vi "3D_to_Pixels.vi"(0 "X_3D":dbl, 5 "Y_3D":dbl, 7 "Z_3D":dbl, 11 "Distance_3D":dbl) -> (4 "X_pixels":dbl, 6 "Y_pixels":dbl, 8 "Z_pixels":dbl, 15 "Distance_pixels":dbl)   [LabVIEW 2011]
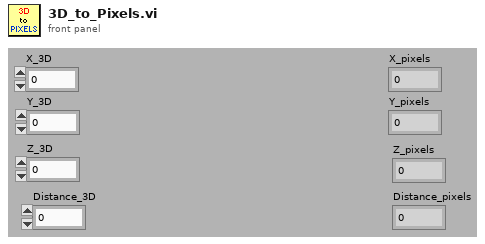
[diagram p1: front panel]
types:
  T1 = typedef "LVAllMonitorsDisplayTypeDef.ctl" = cluster{"Bounds":cluster{"Left":i16, "Top":i16, "Right":i16, "Bottom":i16}, "Depth":i16}[]
  T2 = cluster{"Bounds":cluster{"Left":i16, "Top":i16, "Right":i16, "Bottom":i16}, "Depth":i16}
  T3 = cluster{"Left":i16, "Top":i16, "Right":i16, "Bottom":i16}
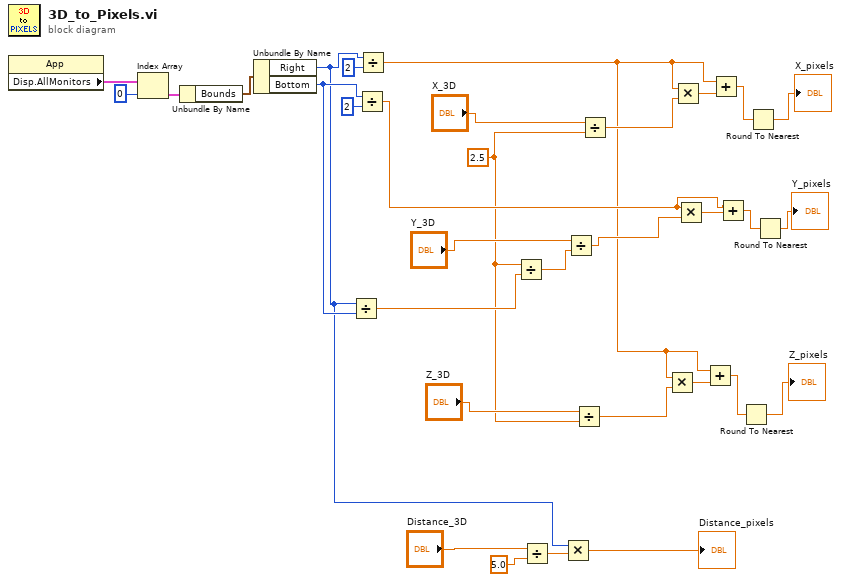
[diagram p0: block diagram]
diagram:
  w8 = 2.5 ("y")
  n1 = property class="App"() -> ("Disp.AllMonitors"=w29:T1)  [unwired: 2 in, 2 out]
  n2 = Index Array(array=w29, index=u16 0 ("Front Panel Window:Monitor")) -> (element=w31:T2)
  n3 = Unbundle By Name(w31) -> ("Bounds"=w28:T3)
  n4 = Unbundle By Name(w28) -> ("Right"=w13:i16, "Bottom"=w24:i16)
  n5 = Divide(x=w13, y=w24) -> (x/y=w22:dbl)
  n6 = Divide(x=w24, y=i16 2) -> (x/y=w17:dbl)
  n7 = Divide(x=w13, y=i16 2) -> (x/y=w9:dbl)
  n8 = Divide(x=w8, y=w22) -> (x/y=w23:dbl)
  n9 = Divide(x="Distance_3D", y=5.0) -> (x/y=w14:dbl)
  n10 = Multiply(x=w13, y=w14) -> (x*y=→"Distance_pixels":dbl)
  n11 = Divide(x="Y_3D", y=w23) -> (x/y=w20:dbl)
  n12 = Divide(x="Z_3D", y=w8) -> (x/y=w11:dbl)
  n13 = Divide(x="X_3D", y=w8) -> (x/y=w21:dbl)
  n14 = Multiply(x=w9, y=w11) -> (x*y=w10:dbl)
  n15 = Multiply(x=w9, y=w21) -> (x*y=w19:dbl)
  n16 = Multiply(x=w17, y=w20) -> (x*y=w18:dbl)
  n17 = Add(x=w9, y=w10) -> (x+y=w3:dbl)
  n18 = Add(x=w9, y=w19) -> (x+y=w7:dbl)
  n19 = Add(x=w17, y=w18) -> (x+y=w5:dbl)
  n20 = Round To Nearest(number=w3) -> (nearest integer value=→"Z_pixels":dbl)
  n21 = Round To Nearest(number=w7) -> (nearest integer value=→"X_pixels":dbl)
  n22 = Round To Nearest(number=w5) -> (nearest integer value=→"Y_pixels":dbl)
